vi "AE-GroupSR_Stats(SubVI).vi"(8 "error in (no error)":errorcluster, 10 "Search Week":i16, 11 "Report Data":T1[](array[typedef])) -> (0 "error out":errorcluster, 3 "Stats Out":T2)   [LabVIEW 2017, in "DS_Lib.lvlib" / "SRReportParser.lvlib"]
uses:
  SRReportParser.lvlib
  TypeDefs/Weekly_SR_Stats.ctl
  Modules/Private Controls/Data Raw.ctl
  Modules/Data Operations.lvlib
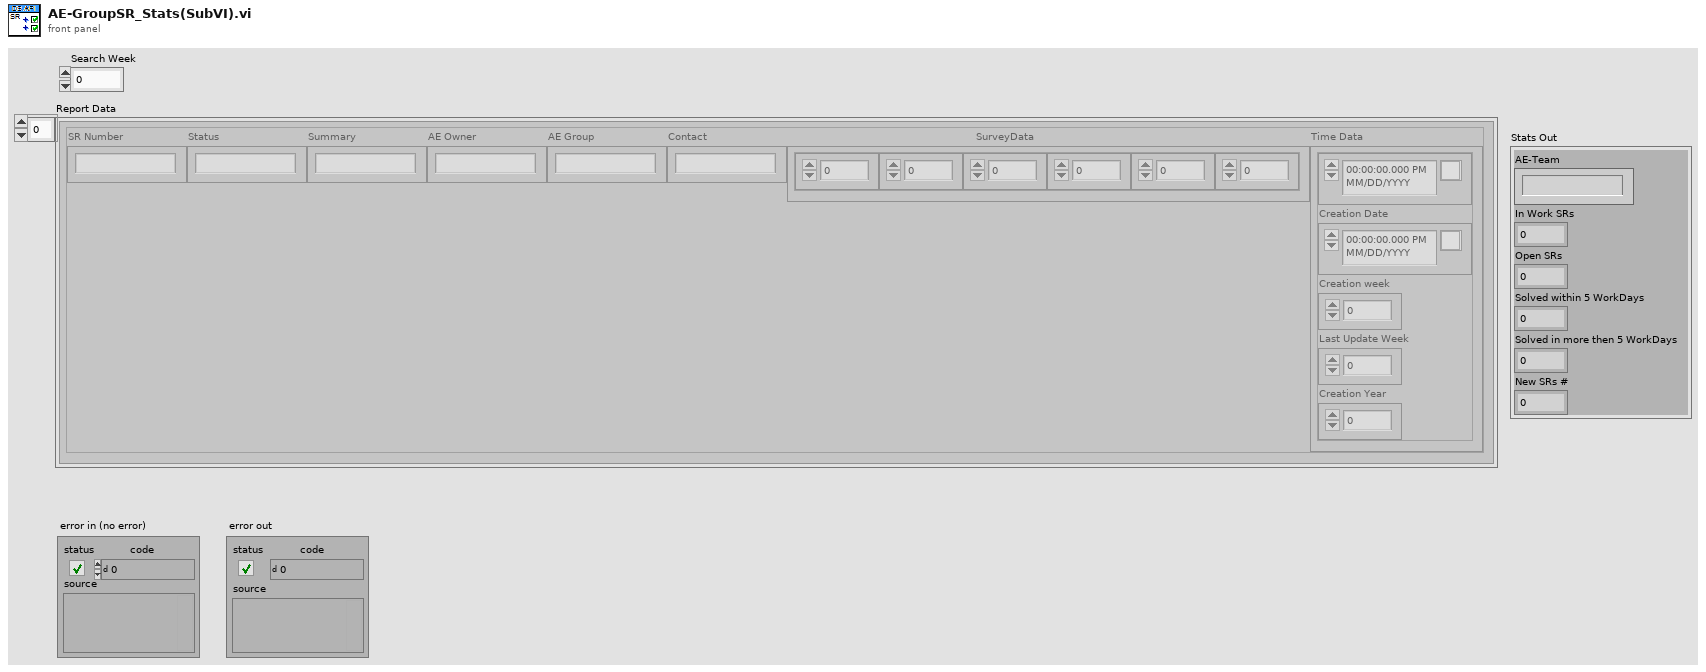
[diagram p1: front panel]
types:
  T1 = typedef "Data Operations.lvlib/Data Raw.ctl" = cluster{"SR Number":string, "Status":string, "Summary":string, "AE Owner":string, "AE Group":string, "Contact":string, "SurveyData":cluster{"Resolution Time":dbl, "Total Satisfaction":dbl, "Response Time":dbl, "Courtesy":dbl, "Problem Solved":dbl, "Level of effort":dbl}, "Time Data":cluster{"Last Update Date":timestamp, "Creation Date":timestamp, "Creation week":i16, "Last Update Week":i16, "Creation Year":i16}}
  T2 = typedef "DS_Lib.lvlib/SRReportParser.lvlib/Weekly_SR_Stats.ctl" = cluster{"AE-Team":string, "In Work SRs":i32, "Open SRs":i32, "Solved within 5 WorkDays":i32, "Solved in more then 5 WorkDays":i32, "New SRs #":i32}
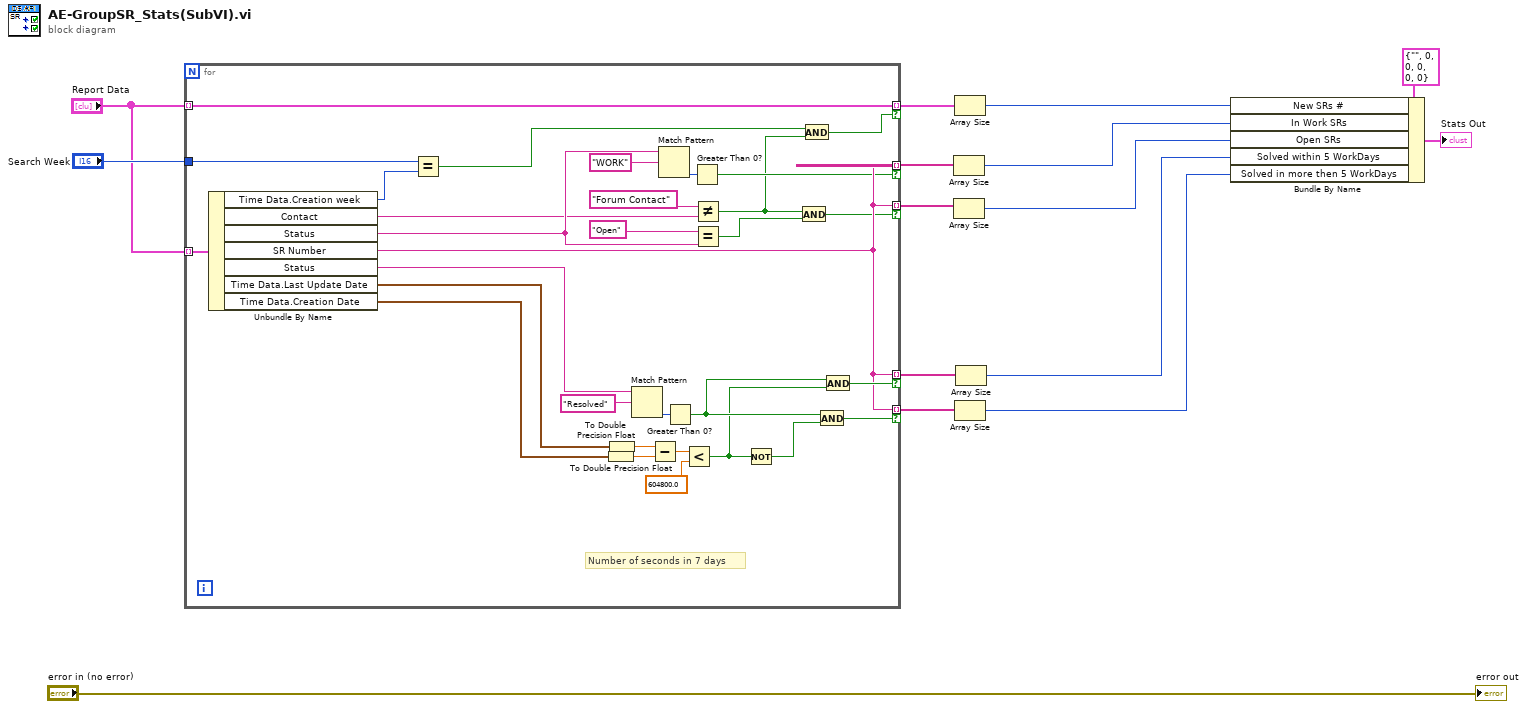
[diagram p0: block diagram]
diagram:
  n1 = for {
    tunnel: "Report Data" -> [w46] mode=indexing
    tunnel: [w31] -> w12 mode=indexing if=w42
    tunnel: [w31] -> w13 mode=indexing if=w35
    tunnel: [w31] -> w14 mode=indexing if=w28
    tunnel: [w31] -> w15 mode=indexing if=w21
    tunnel: "Report Data" -> [w23] mode=indexing
    tunnel: [w23] -> w4 mode=indexing if=w20
    tunnel: "Search Week" -> [w17]
    # "Number of seconds in 7 days"
    n2 = Unbundle By Name(w46) -> ("Time Data.Creation week"=w18:i16, "Contact"=w24:string, "Status"=w25:string, "SR Number"=w31:string, "Status"=w45:string, "Time Data.Last Update Date"=w41:timestamp, "Time Data.Creation Date"=w40:timestamp)
    n3 = Equal?(x=w17, y=w18) -> (x = y?=w16:bool)
    n4 = To Double Precision Float(number=w40) -> (double precision float=w39:dbl)
    n5 = To Double Precision Float(number=w41) -> (double precision float=w38:dbl)
    n6 = Match Pattern(string=w45, regular expression="Resolved" ("y")) -> (offset past match=w43:i32)  [unwired: 1 in, 3 out]
    n7 = Subtract(x=w38, y=w39) -> (x-y=w32:dbl)
    n8 = Match Pattern(string=w25, regular expression="WORK" ("y")) -> (offset past match=w30:i32)  [unwired: 1 in, 3 out]
    n9 = Greater Than 0?(x=w43) -> (x > 0?=w34:bool)
    n10 = Less?(x=w32, y=604800.0) -> (x < y?=w33:bool)
    n11 = Greater Than 0?(x=w30) -> (x > 0?=w21:bool)
    n12 = Not Equal?(x="Forum Contact" ("y"), y=w24) -> (x != y?=w19:bool)
    n13 = Equal?(x="Open" ("y"), y=w25) -> (x = y?=w22:bool)
    n14 = Not(x=w33) -> (.not. x?=w36:bool)
    n15 = And(x=w19, y=w22) -> (x .and. y?=w28:bool)
    n16 = And(x=w16, y=w19) -> (x .and. y?=w20:bool)
    n17 = And(x=w34, y=w36) -> (x .and. y?=w35:bool)
    n18 = And(x=w34, y=w33) -> (x .and. y?=w42:bool)
  }
  n19 = Array Size(array=w15) -> (size(s)=w10:i32)
  n20 = Array Size(array=w14) -> (size(s)=w9:i32)
  n21 = Array Size(array=w4) -> (size(s)=w3:i32)
  n22 = Array Size(array=w13) -> (size(s)=w7:i32)
  n23 = Array Size(array=w12) -> (size(s)=w8:i32)
  n24 = Bundle By Name(cluster=T2 {"AE-Team"="", "In Work SRs"=0, "Open SRs"=0, "Solved within 5 WorkDays"=0, "Solved in more then 5 WorkDays"=0, "New SRs #"=0}, "New SRs #"=w3, "In Work SRs"=w10, "Open SRs"=w9, "Solved within 5 WorkDays"=w8, "Solved in more then 5 WorkDays"=w7) -> (→"Stats Out":T2)
  "error out" <- "error in (no error)"
